vi "VIP Version.vi"(0 "Home version":bool, 1 "Force Check(F)":bool, 11 "error in":errorcluster) -> (2 "Version":T2, 4 "VIP version":string, 6 "Check Version":bool, 8 "Latest":T1, 10 "Found":bool, 15 "error out":errorcluster)   [LabVIEW 2014, in "Raspberry Pi Compatible Compiler for LabVIEW.lvlib"]
uses:
  Raspberry Pi Compatible Compiler for LabVIEW.lvlib
  RasPi_Services/Download/RuntimeVersion.ctl
  GitHub/TypeDefs/GitHubContents_TD.ctl
  GitHub/TypeDefs/GitHubCheckTypeTD.ctl
  Compile and Download App/Custom Controls/Local Setup Parameters.ctl
  GitHub/GitHub API.lvlib
  RasPi_Services/Download/RasPiDownloader.lvlib
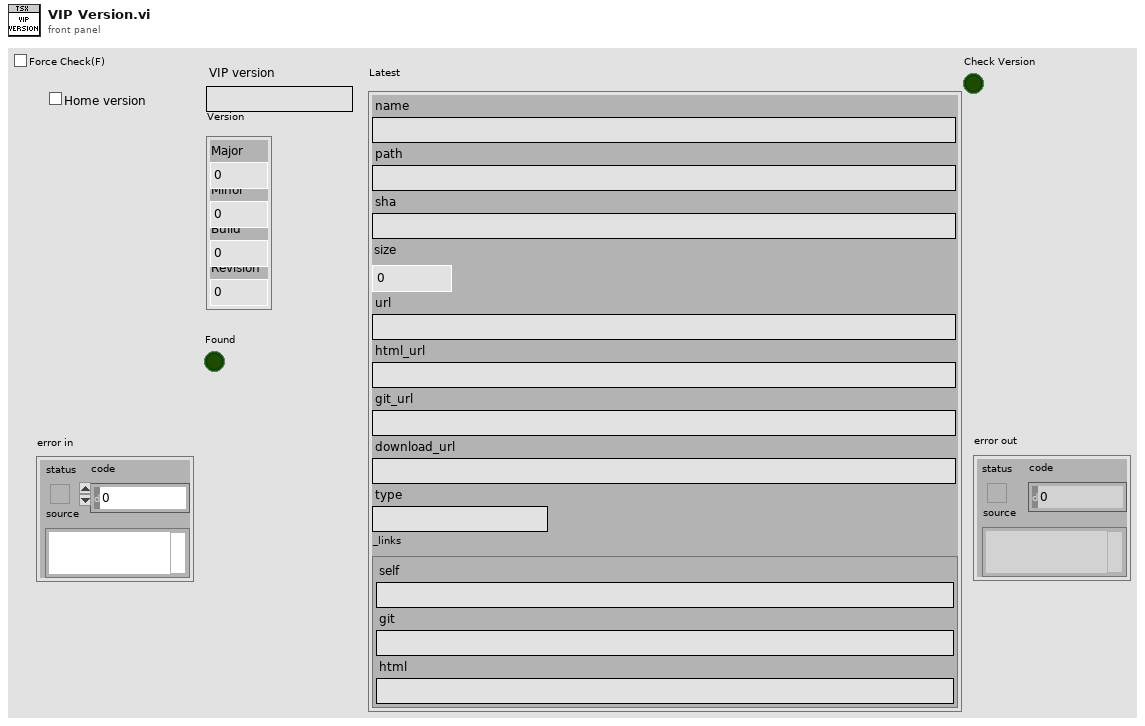
[diagram p1: front panel]
types:
  T1 = typedef "Raspberry Pi Compatible Compiler for LabVIEW.lvlib/GitHub API.lvlib/GitHubContents_TD.ctl" = cluster{"name":string, "path":string, "sha":string, "size":dbl, "url":string, "html_url":string, "git_url":string, "download_url":string, "type":string, "_links":cluster{"self":string, "git":string, "html":string}}
  T2 = typedef "Raspberry Pi Compatible Compiler for LabVIEW.lvlib/RasPiDownloader.lvlib/RuntimeVersion.ctl" = cluster{"Major":i32, "Minor":i32, "Build":i32, "Revision":i32}
  T3 = typedef "Raspberry Pi Compatible Compiler for LabVIEW.lvlib/GitHub API.lvlib/GitHubCheckTypeTD.ctl" = enum16{"runtime", "VIPM Home Version", "VIPM Standard Version"}
  T4 = typedef "Raspberry Pi Compatible Compiler for LabVIEW.lvlib/Local Setup Parameters.ctl" = enum16{"Add Last VI", "Read Last VI", "Add Board IP", "Remove Board IP", "Read All Board IP", "Add Runtime Version", "Read Runtime Version", "Add Package Version", "Read Package Version", "Add VIPCheck Time", "Read VIPCheck Time"}
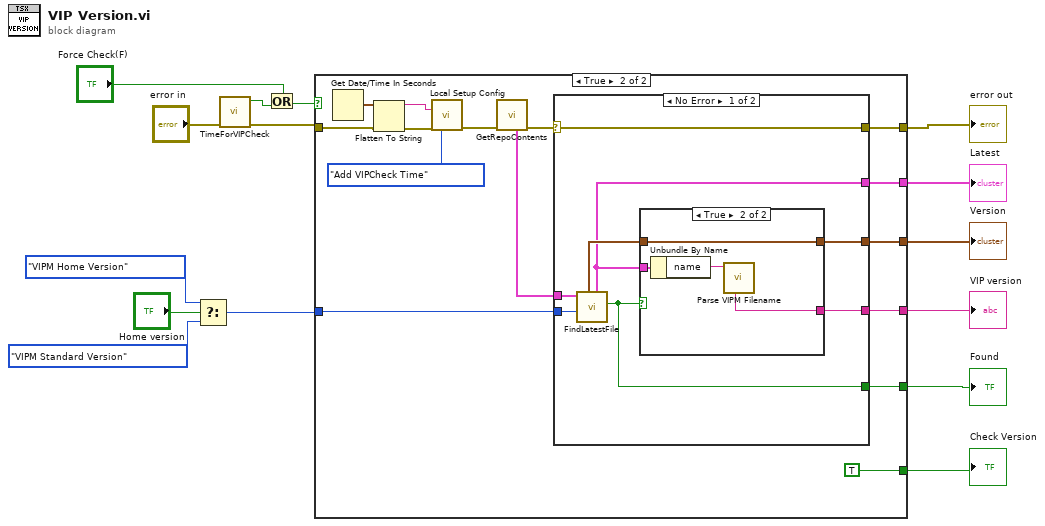
[diagram p0: block diagram]
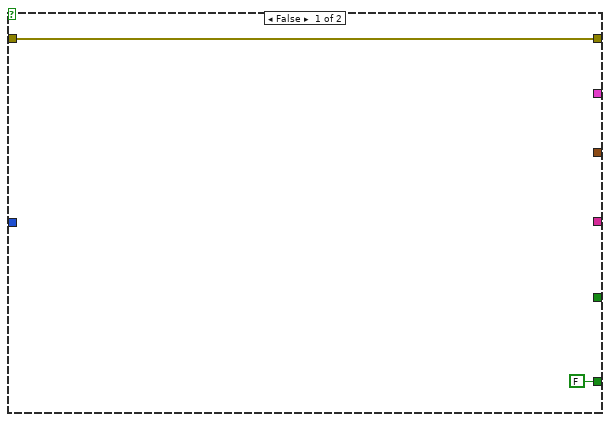
[diagram p2: hidden frame]
diagram:
  n1 = Select(t=GitHubCheckTypeTD."VIPM Home Version" ("Check Type"), s="Home version", f=GitHubCheckTypeTD."VIPM Standard Version" ("Check Type")) -> (s? t:f=w12:T3)
  n2 = call "TimeForVIPCheck.vi"("error in (no error)"="error in") -> ("error out"=w4:errorcluster, "Check VIP?"=w3:bool)  [unwired: 9 in]
  n3 = Or(x="Force Check(F)", y=w3) -> (x .or. y?=w2:bool)
  n4 = case shown="True" w2 {
    tunnel: w4 -> [w16 w21]
    tunnel: w12 -> [_ w31]
    tunnel: [w16 w29] -> w11
    tunnel: [_ w28] -> w10
    tunnel: [_ w27] -> w9
    tunnel: [_ w26] -> w8
    tunnel: [_ w25] -> w7
    tunnel: [FALSE TRUE] -> w6
    frame False {
    }
    frame True {
      n5 = Get Date/Time In Seconds() -> (seconds since 1Jan1904=w20:timestamp)
      n6 = Flatten To String(anything=w20, error in (no error)=w21) -> (data string=w18:string, error out=w19:errorcluster)  [unwired: 2 in, 1 out]
      n7 = call "Local Setup Config.vi"("Local Setup Param"=Local_Setup_Parameters."Add VIPCheck Time", "KeyValue"=w18, "error in"=w19) -> ("error out"=w23:errorcluster)  [unwired: 9 in, 3 out]
      n8 = call "GetRepoContents.vi"("error in"=w23) -> ("error out"=w30:errorcluster, "Contents"=w32:T1[])  [unwired: 7 in]
      n9 = case shown="No Error" w30 {
        selector: w30 -> [w39 w45]
        tunnel: w32 -> [w35 _]
        tunnel: w31 -> [w40 _]
        tunnel: [w39 w45] -> w29
        tunnel: [w38 _] -> w28
        tunnel: [w36 _] -> w27
        tunnel: [w33 _] -> w25
        tunnel: [w34 _] -> w26
        frame No Error {
          n10 = call "FindLatestFile.vi"("Check Type"=w40, "Contents"=w35) -> ("Found"=w34:bool, "Latest runtime"=w33:T1, "Version"=w37:T2)  [unwired: 5 in]
          n11 = case shown="True" w34 {
            tunnel: w33 -> [_ w44]
            tunnel: [_ w42] -> w38
            tunnel: [_ w41] -> w36
            tunnel: w37 -> [_ w41]
            frame False {
            }
            frame True {
              n12 = Unbundle By Name(w44) -> ("name"=w43:string)
              n13 = call "Parse VIPM Filename.vi"("Filename"=w43) -> ("version"=w42:string)  [unwired: 7 in, 1 out]
            }
          }
        }
        frame Error {
        }
      }
    }
  }
  "error out" <- w11
  "VIP version" <- w10
  "Version" <- w9
  "Found" <- w8
  "Latest" <- w7
  "Check Version" <- w6
